vi "Test.vi"() -> ()   [LabVIEW 2018]
doc: "This VI is called when test mode begins, and will automatically be terminated when it ends. You can add manual or automatic tests and invoke them from the dashboard."
uses:
  <vilib>/Rock Robotics/WPI/ThirdParty/Phoenix-LabVIEW/Motor Controller/Controls/CTRE_Phoenix_MotorControl_ControlMode.ctl
  Infrastructure/Constants.vi
  <vilib>/Rock Robotics/WPI/ThirdParty/Phoenix-LabVIEW/Motor Controller/Get/CTRE_Phoenix_MotorController_GetSelectedSensorData.vi
panel:
  in  "ZeroSensor":bool
  in  "Output":dbl
  in  "Control Mode":T1 items=["PercentOutput"=0, "Position"=1, "Velocity"=2, "Current"=3, "Follower"=5, "MotionProfile"=6, "MotionMagic"=7, "MotionProfileArc"=10, "Disabled"=15]
  out "Velocity":i32(graph)
  out "Position":i32(graph)
  in  "System To Tune":T2(ring)
  in  "Running From Main to Tune":bool
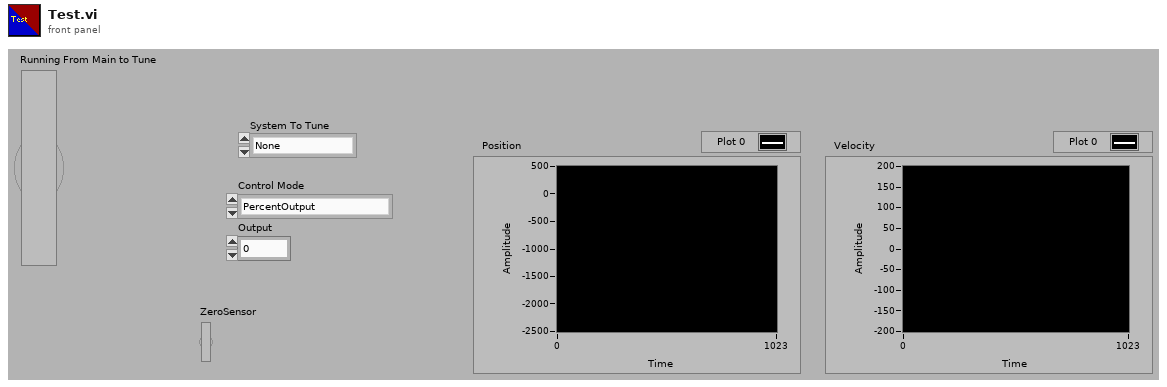
[diagram p1: front panel]
types:
  T1 = typedef "CTRE_Phoenix_MotorControl_ControlMode.ctl" = u16
  T2 = enum16{"None", "LeftDrive", "RightDrive", "4bar", "HPIntake"}
  T3 = enum8{"Enabled", "Disabled", "Disabled and Grayed Out"}
  T4 = cluster{"Cruise Velocity":i32, "Acceleration":i32}
  T5 = cluster{"P":dbl, "I":dbl, "D":dbl, "F":dbl, "I Zone":dbl}
  T6 = typedef "WPI_MotorControlDeviceRef.ctl" = cluster{"DeviceStatus":errorcluster, "Type":T7, "PWM":cluster{"PWM Channel":T8, "DeadBand":T9}, "CAN":cluster{"Device Number":u8, "SetOutput VI Ref":variant, "GetOutput VI Ref":variant, "Enable VI Ref":variant, "Disable VI Ref":variant, "Data":variant}, "Invert":bool, "DIO PWM":cluster{"PWM \"Enable\" Channel":T8, "DIOChannel":T10, "PWM Rate":dbl}}
  T7 = typedef "WPI_MotorControlType.ctl" = enum16{"PWM", "CAN", "DIO PWM"}
  T8 = typedef "FPGA_DIOPWMChannel.ctl" = enum8{"PWM 0", "PWM 1", "PWM 2", "PWM 3", "PWM 4", "PWM 5", "PWM 6", "PWM 7", "PWM 8", "PWM 9", "PWM MXP 0", "PWM MXP 1", "PWM MXP 2", "PWM MXP 3", "PWM MXP 4", "PWM MXP 5", "PWM MXP 6", "PWM MXP 7", "PWM MXP 8", "PWM MXP 9", "Invalid"}
  T9 = typedef "WPI_PWMDeadband.ctl" = cluster{"Name":string, "maxPositivePwm":i32, "minPositivePwm":i32, "centerPwm":i32, "maxNegativePwm":i32, "minNegativePwm":i32, "angularRange":u16}
  T10 = typedef "FPGA_DIOChannel.ctl" = enum8{"DIO 0", "DIO 1", "DIO 2", "DIO 3", "DIO 4", "DIO 5", "DIO 6", "DIO 7", "DIO 8", "DIO 9", "DIO MXP 0", "DIO MXP 1", "DIO MXP 2", "DIO MXP 3", "DIO MXP 4", "DIO MXP 5", "DIO MXP 6", "DIO MXP 7", "DIO MXP 8", "DIO MXP 9", "DIO MXP 10", "DIO MXP 11", "DIO MXP 12", "DIO MXP 13", "DIO MXP 14", "DIO MXP 15", "SPI Port CS1", "SPI Port CS2", "SPI Port CS3", "SPI Port MISO", "SPI Port MOSI", "Invalid"}
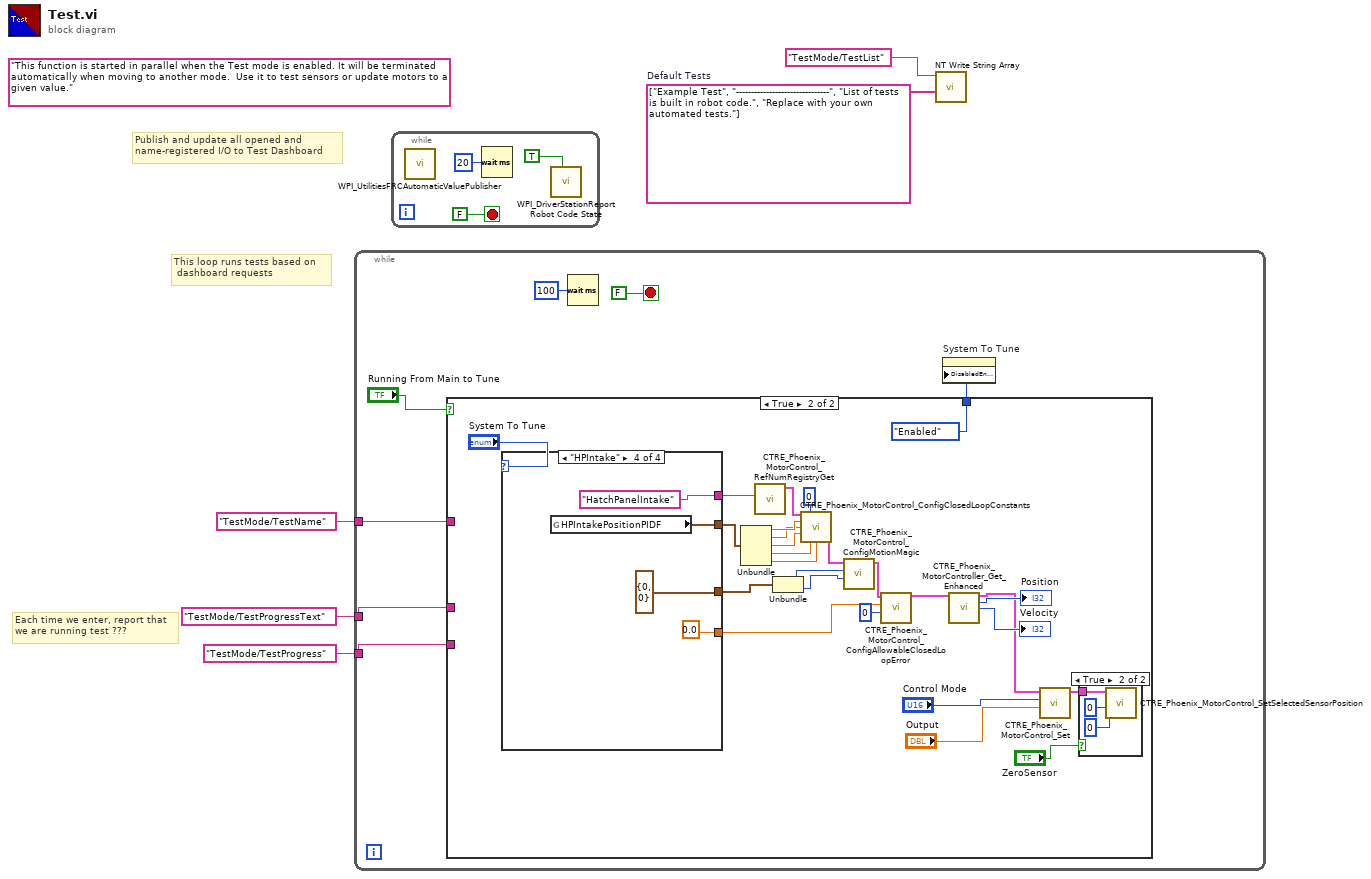
[diagram p0: block diagram]
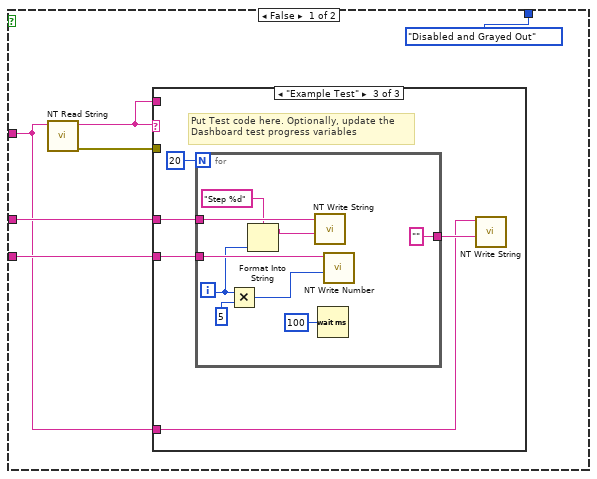
[diagram p2: hidden frame]
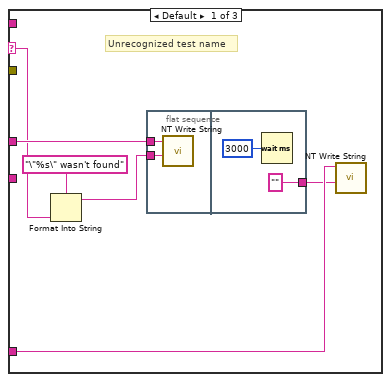
[diagram p3: hidden frame]
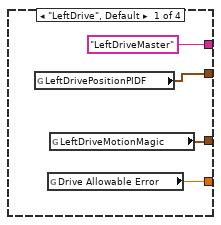
[diagram p6: hidden frame]
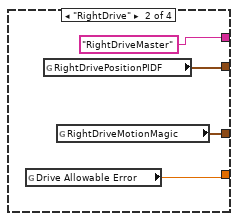
[diagram p7: hidden frame]
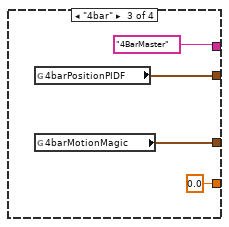
[diagram p8: hidden frame]
diagram:
  w2 = string[] ["Example Test", "-------------------------------", "List of tests is built in robot code.", "Replace with your own automated tests."]  # Default Tests
  (unwired) "This function is started in parallel when the Test mode is enabled. It will be terminated automatically when moving to another mode.  Use it to test sensors or update motors to a given value."
  # "This loop runs tests based on \n dashboard requests"
  # "Publish and update all opened and\nname-registered I/O to Test Dashboard"
  # "Each time we enter, report that\nwe are running test ???"
  n1 = while {
    tunnel: "TestMode/TestName" ("Name") -> [w8]
    tunnel: "TestMode/TestProgressText" ("Name") -> [w10]
    tunnel: "TestMode/TestProgress" ("Name") -> [w9]
    stop <- FALSE stop-if-true
    n2 = case shown="True" "Running From Main to Tune" {
      tunnel: w10 -> [w18 _]
      tunnel: w9 -> [w17 _]
      tunnel: w8 -> [w15 _]
      tunnel: [T3."Disabled and Grayed Out" ("Disabled") T3."Enabled" ("Disabled")] -> w6
      frame False {
        n3 = call <vilib>:"NT Read String.vi"("Name"=w15) -> ("error out"=w14:errorcluster, "String"=w16:string)  [unwired: 9 in]
        n4 = case shown="\"Example Test\"" w16 {
          selector: w16 -> [w23 _ _]
          tunnel: w15 -> [w20 _ w29]
          tunnel: w18 -> [w24 _ w32]
          tunnel: w17 -> [_ _ w33]
          tunnel: w16 -> [_ _ _]
          tunnel: w14 -> [_ _ _]
          frame Default {
            # "Unrecognized test name"
            n5 = Format Into String(format string="\"%s\" wasn't found" ("Name"), w23) -> (resulting string=w22:string)  [unwired: 2 in, 1 out]
            n6 = flat-sequence {
              tunnel: w24 -> [w25]
              tunnel: w22 -> [w26]
              tunnel: ["" ("Name")] -> w19
              frame #0 {
                n7 = call <vilib>:"NT Write String.vi"("String"=w26, "Name"=w25) -> ()  [unwired: 9 in, 1 out]
              }
              frame #1 {
                n8 = Wait (ms)(milliseconds to wait=u32 3000) -> ()  [unwired: 1 out]
              }
            }
            n9 = call <vilib>:"NT Write String.vi"("String"=w19, "Name"=w20) -> ()  [unwired: 9 in, 1 out]
          }
          frame "" {
            # "No test to run"
          }
          frame "Example Test" {
            # "Put Test code here. Optionally, update the\nDashboard test progress variables"
            n10 = for {
              N: 20 -> [_]
              tunnel: w33 -> [w42]
              tunnel: w32 -> [w40]
              tunnel: ["" ("String")] -> w30
              i -> [w37]
              n11 = Multiply(x=w37, y=u32 5 ("milliseconds to wait")) -> (x*y=w38:u32)
              n12 = Format Into String(format string="Step %d", w37) -> (resulting string=w35:string)  [unwired: 2 in, 1 out]
              n13 = call <vilib>:"NT Write String.vi"("String"=w35, "Name"=w40) -> ()  [unwired: 9 in, 1 out]
              n14 = Wait (ms)(milliseconds to wait=u32 100) -> ()  [unwired: 1 out]
              n15 = call <vilib>:"NT Write Number.vi"("Numeric"=w38, "Name"=w42) -> ()  [unwired: 9 in, 1 out]
            }
            n16 = call <vilib>:"NT Write String.vi"("String"=w30, "Name"=w29) -> ()  [unwired: 9 in, 1 out]
          }
        }
      }
      frame True {
        n17 = case shown="\"HPIntake\"" "System To Tune" {
          tunnel: ["LeftDriveMaster" ("refnum name") "RightDriveMaster" ("refnum name") "4BarMaster" ("refnum name") "HatchPanelIntake" ("refnum name")] -> w66
          tunnel: [w74 w78 w82 w86] -> w61
          tunnel: [w73 w77 w81 T4 {"Cruise Velocity"=0, "Acceleration"=0} ("4barMotionMagic")] -> w55
          tunnel: [w72 w76 0.0 ("Drive Allowable Error") 0.0 ("Drive Allowable Error")] -> w52
          frame "LeftDrive", Default {
            n18 = global read "Constants.vi" "LeftDrivePositionPIDF"() -> (w74:T5)
            n19 = global read "Constants.vi" "Drive Allowable Error"() -> (w72:dbl)
            n20 = global read "Constants.vi" "LeftDriveMotionMagic"() -> (w73:T4)
          }
          frame "RightDrive" {
            n21 = global read "Constants.vi" "Drive Allowable Error"() -> (w76:dbl)
            n22 = global read "Constants.vi" "RightDrivePositionPIDF"() -> (w78:T5)
            n23 = global read "Constants.vi" "RightDriveMotionMagic"() -> (w77:T4)
          }
          frame "4bar" {
            n24 = global read "Constants.vi" "4barPositionPIDF"() -> (w82:T5)
            n25 = global read "Constants.vi" "4barMotionMagic"() -> (w81:T4)
          }
          frame "HPIntake" {
            n26 = global read "Constants.vi" "HPIntakePositionPIDF"() -> (w86:T5)
          }
        }
        n27 = Unbundle(w61) -> ("P"=w60:dbl, "I"=w59:dbl, "D"=w58:dbl, "F"=w57:dbl, "I Zone"=w56:dbl)
        n28 = call <vilib>:"CTRE_Phoenix_MotorControl_RefNumRegistryGet.vi"("refnum name"=w66) -> ("PhoenixMotorControlDevRef"=w65:T6)  [unwired: 9 in, 1 out]
        n29 = Unbundle(w55) -> ("Cruise Velocity"=w54:i32, "Acceleration"=w53:i32)
        n30 = call <vilib>:"CTRE_Phoenix_MotorControl_ConfigClosedLoopConstants.vi"("PhoenixMotorControlDevRef"=w65, "slotIdx"=0, "P"=w60, "I"=w59, "D"=w58, "F"=w57, "I Zone"=w56) -> ("PhoenixMotorControlDevRef"=w64:T6)  [unwired: 7 in, 1 out]
        n31 = call <vilib>:"CTRE_Phoenix_MotorControl_ConfigMotionMagic.vi"("Acceleration"=w53, "Cruise Velocity"=w54, "PhoenixMotorControlDevRef"=w64) -> ("PhoenixMotorControlDevRef"=w63:T6)  [unwired: 7 in, 1 out]
        n32 = call <vilib>:"CTRE_Phoenix_MotorControl_ConfigAllowableClosedLoopError.vi"("slotIdx"=u32 0, "allowableClosedLoopError"=w52, "PhoenixMotorControlDevRef"=w63) -> ("PhoenixMotorControlDevRef"=w50:T6)  [unwired: 7 in, 1 out]
        n33 = call-poly <vilib>:"CTRE_Phoenix_MotorController_Get_Enhanced.vi"("PhoenixMotorControlDevRef"=w50) -> ("PhoenixMotorControlDevRef"=w47:T6, "Position (Raw Sensor Units)"=→"Position":i32, "Velocity (Raw Sensor Units per 100 ms)"=→"Velocity":i32)  [unwired: 11 in, 1 out]
        n34 = call <vilib>:"CTRE_Phoenix_MotorControl_Set.vi"("Output"="Output", "Control Mode"="Control Mode", "PhoenixMotorControlDevRef"=w47) -> ("PhoenixMotorControlDevRef"=w44:T6)  [unwired: 7 in, 1 out]
        n35 = case shown="True" "ZeroSensor" {
          tunnel: w44 -> [_ w71]
          frame False {
          }
          frame True {
            n36 = call <vilib>:"CTRE_Phoenix_MotorControl_SetSelectedSensorPosition.vi"("pidLoopIdx"=u32 0, "New Sensor Position"=0, "PhoenixMotorControlDevRef"=w71) -> ()  [unwired: 7 in, 2 out]
          }
        }
      }
    }
    n37 = Wait (ms)(milliseconds to wait=u32 100) -> ()  [unwired: 1 out]
    n38 = property on="System To Tune" class="Enum (strict)"("DisabledEnum"=w6) -> ()  [unwired: 2 in, 2 out]
  }
  n39 = while {
    stop <- FALSE stop-if-true
    n40 = call <vilib>:"WPI_UtilitiesFRCAutomaticValuePublisher.vi"() -> ()  [unwired: 12 in]
    n41 = Wait (ms)(milliseconds to wait=u32 20) -> ()  [unwired: 1 out]
    n42 = call <vilib>:"WPI_DriverStationReport Robot Code State.vi"("Test"=TRUE ("Autonomous")) -> ()  [unwired: 10 in, 1 out]
  }
  n43 = call <vilib>:"NT Write String Array.vi"("String Array"=w2, "Name"="TestMode/TestList") -> ()  [unwired: 9 in, 1 out]
